vi "basic - Transmit UDP Sampling.vi"() -> ()   [LabVIEW 2020]
uses:
  _controls/comm_computedMAC-IP.ctl
  _controls/comm_udp_tx.ctl
  _controls/comm_config_vl_tx.ctl
  _polimorphicInstances/session/Fdx Create Session (Tx-UDP Port-Oriented).vi
  bsp/AFDX_Transmit/Fdx Create Tx VL.vi
  _polimorphicInstances/udpPort/Fdx Create UDP Port (TX-CommPort).vi
  _polimorphicInstances/control/Fdx Start (Tx).vi
  _polimorphicInstances/control/Fdx Stop (Tx).vi
  _polimorphicInstances/session/Fdx Close Session (Port).vi
  AIM664LV.lvlib
panel:
  out "Duplicated":bool
  in  "VL Config":T1={"VlId"=60, "NumOfSubVl"=2, "rate ms [Bag]"=128, "domainID"=1, "sideID"=1, "locationID"=1, "interfaceID"=1, "NetSelect"=3, "Skew"=0, "MaxFrameLength"=1000, "FrameBufferSize"=0} {"NetSelect" items=["FDX_TX_FRAME_DLY_A"=0, "FDX_TX_FRAME_DLY_B"=1, "FDX_TX_FRAME_BOTH "=3, "FDX_TX_FRAME_ONLY_A"=4, "FDX_TX_FRAME_ONLY_B "=5]; "interfaceID" format="%.0b"}
  in  "CommPort Config":T2[](array[typedef])=[{"PortType"=enum."FDX_UDP_SAMPLING", "partitionID"=1, "SubVlId"=1, "UdpSrcPort"=1, "UdpDstPort"=1, "SampleRateMs"=128.0, "UdpNumBufMessages"=0, "UdpMaxMessageSize"=1000}, {"PortType"=enum."FDX_UDP_SAMPLING", "partitionID"=1, "SubVlId"=2, "UdpSrcPort"=2, "UdpDstPort"=2, "SampleRateMs"=128.0, "UdpNumBufMessages"=0, "UdpMaxMessageSize"=1000}]
  in  "millisecond multiple":u32=128
  in  "PortMap":u32
  out "IndexCycleCount":u32[](array[numeric])
  out "MsgCount":u32[](array[numeric])
  out "CurrentIndex":u32[](array[numeric])
  out "BytesWritten":u32[](array[numeric])
  in  "Port":u32
  in  "Board":u32
  out "current time":timestamp=timestamp(3677762637.591913 s since 1904-01-01)
  out "current irig time":T3={"SignOut"=40, "DayOut"=1, "HourOut"=1, "MinOut"=28, "SecondOut"=39, "MilliSecOut"=539, "MicroSecOut"=300, "NanoSecOut"=0, "InfoOut"=0, "Mode"=3}
  out "CommPort Addresses":T4[](array[typedef]) {"MACsrc" format="%.0x"}
  out "Data to be sent":u8[](array[numeric])=[255, 255, 255, 255, 255, 255, 255, 255, 255, 255, 255, 255, 255, 255, 255, 255, 255, 255, 255, 255, 255, 255, 255, 255, 255, 255, 255, 255, 255, 255, 255, 255, 255, 255, 255, 255, 255, 255, 255, 255, 255, 255, 255, 255, 255, 255, 255, 255, 255, 255, 255, 255, 255, 255, 255, 255, 255, 255, 255, 255, 255, 255, 255, 255, 255, 255, 255, 255, 255, 255, 255, 255, 255, 255, 255, 255, 255, 255, 255, 255, 255, 255, 255, 255, 255, 255, 255, 255, 255, 255, 255, 255, 255, 255, 255, 255, 255, 255, 255, 170] format="%.0x"
  in  "stop":bool
  out "PortInitOut":T5={"PortConfig"=0, "PortUsed"=1, "GlobalMemFree"=0, "SharedMemFree"=0} {"PortConfig" items=["FDX_SINGLE", "FDX_REDUNDANT"]}
  out "error out":errorcluster
  # "ARINC 664 - Transmit UDP - Sampling Port"
  # "Overview: Setup the board to transmit package as UDP using Sampling Port.\n\nRequirement: One AIM ARINC-664 board with installed AIM ARINC 664 BSP.\nRestrictions: None.\nInstruction:\n1. Select the Board ID (0 if you have only one board in your system) and the port number. If you want to validate between two ports in one device, you can use tx board and Rx Board\n2. Run the VI.\n3. See the result in Current IRIG Time"
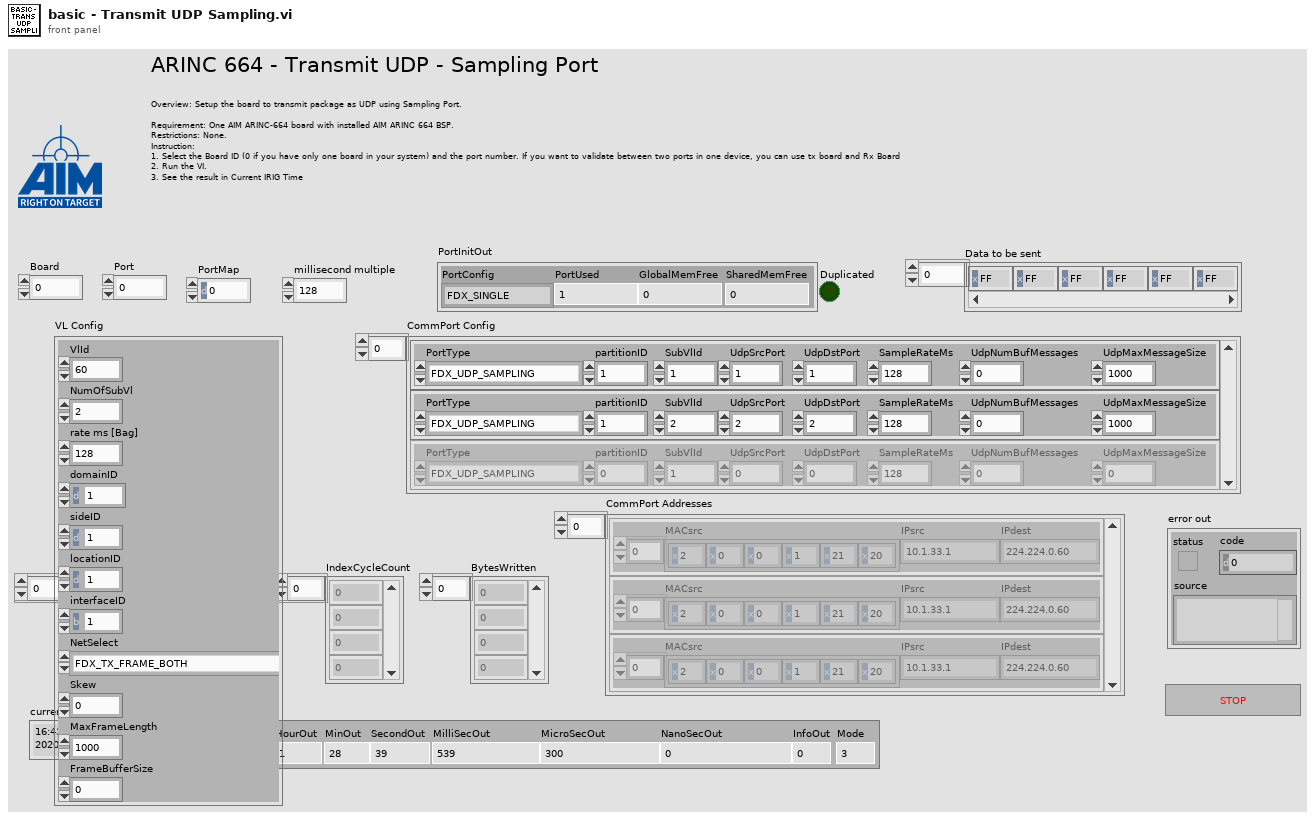
[diagram p1: front panel]
types:
  T1 = typedef "AIM664LV.lvlib/comm_config_vl_tx.ctl" = cluster{"VlId":u16, "NumOfSubVl":u16, "rate ms [Bag]":u32, "domainID":u8, "sideID":u8, "locationID":u8, "interfaceID":u8, "NetSelect":u32, "Skew":u32, "MaxFrameLength":u32, "FrameBufferSize":u32}
  T2 = typedef "AIM664LV.lvlib/comm_udp_tx.ctl" = cluster{"PortType":enum16{"FDX_UDP_SAMPLING", "FDX_UDP_QUEUING"}, "partitionID":u8, "SubVlId":u8, "UdpSrcPort":u16, "UdpDstPort":u16, "SampleRateMs":dbl, "UdpNumBufMessages":u32, "UdpMaxMessageSize":u32}
  T3 = cluster{"SignOut":i32, "DayOut":u32, "HourOut":u32, "MinOut":u32, "SecondOut":u32, "MilliSecOut":u32, "MicroSecOut":u32, "NanoSecOut":u32, "InfoOut":u32, "Mode":u32}
  T4 = typedef "AIM664LV.lvlib/comm_computedMAC-IP.ctl" = cluster{"MACsrc":u8[], "IPsrc":string, "IPdest":string}
  T5 = cluster{"PortConfig":u32, "PortUsed":u32, "GlobalMemFree":u32, "SharedMemFree":u32}
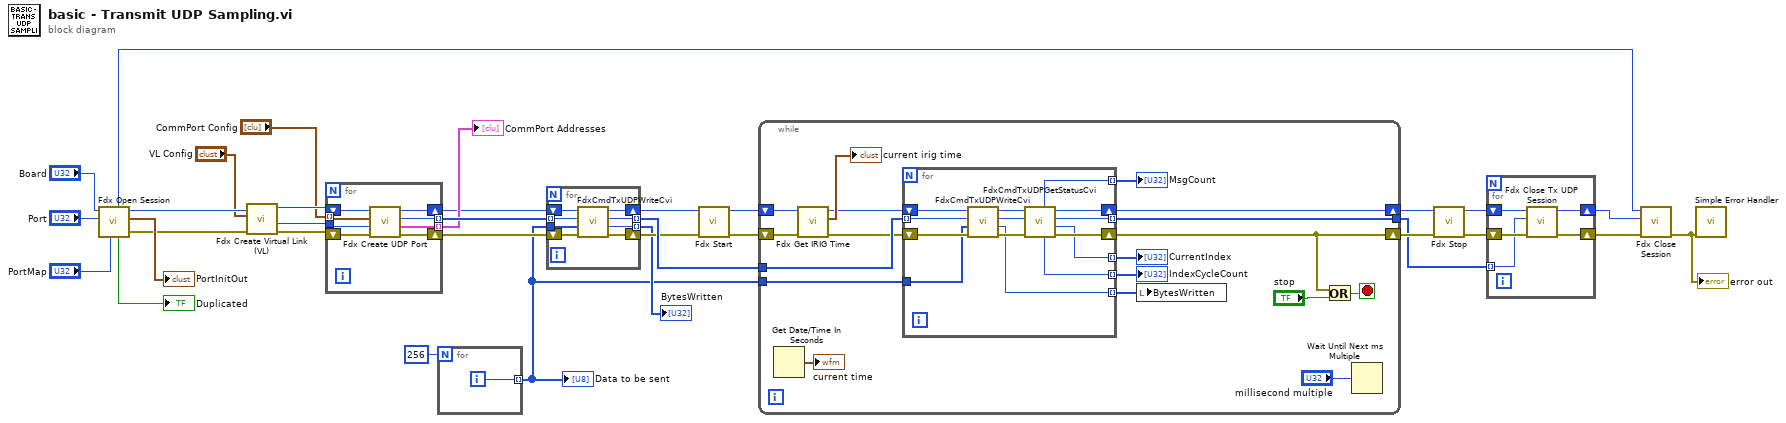
[diagram p0: block diagram]
diagram:
  n1 = call-poly "Fdx Open Session.vi"("PortMap"="PortMap", "port"="Port", "board"="Board") -> ("error out"=w16:errorcluster, "PortInitOut"=→"PortInitOut":T5, "port handle out"=w17:u32, "Duplicated"=→"Duplicated":bool, "InstrumentHandle_board out"=w1:u32)  [unwired: 4 in]
  n2 = call-poly "Fdx Create Virtual Link (VL).vi"("error in (no error)"=w16, "VL Config"="VL Config", "InstrumentHandle in"=w17) -> ("error out"=w14:errorcluster, "VlId"=w13:u16, "InstrumentHandle out"=w15:u32)  [unwired: 6 in]
  n3 = for {
    tunnel: [w40] -> w32 mode=indexing
    tunnel: [w37] -> w29 mode=indexing
    shift-right: [w36] -> w8
    shift-left: w15 -> [w41]
    shift-right: [w39] -> w30
    shift-left: w14 -> [w38]
    tunnel: w13 -> [w35]
    tunnel: "CommPort Config" -> [w34] mode=indexing
    n4 = call-poly "Fdx Create UDP Port.vi"("error in"=w38, "VlId"=w35, "CommPort Config"=w34, "port handle in"=w41) -> ("error out"=w39:errorcluster, "computedAddresses"=w37:T4, "commPort handle out"=w40:u32, "port handle out"=w36:u32)  [unwired: 4 in]
  }
  "CommPort Addresses" <- w29
  n5 = for {
    N: 256 -> [_]
    tunnel: [w42] -> w2 mode=indexing
    i -> [w42]
  }
  "Data to be sent" <- w2
  n6 = for {
    tunnel: w2 -> [w46]
    tunnel: [w48] -> w19 mode=indexing
    shift-right: [w49] -> w27
    shift-left: w30 -> [w50]
    tunnel: w32 -> [w47] mode=indexing
    tunnel: [w43] -> w31 mode=indexing
    shift-right: [w44] -> w7
    shift-left: w8 -> [w45]
    n7 = call "FdxCmdTxUDPWriteCvi.vi"("error in"=w50, "Data"=w46, "UdpHandle"=w47, "InstrumentHandle"=w45) -> ("error out"=w49:errorcluster, "BytesWritten"=w48:u32, "UdpHandleOut"=w43:u32, "InstrumentHandle"=w44:u32)  [unwired: 4 in]
  }
  "BytesWritten" <- w19
  n8 = call-poly "Fdx Start.vi"("error in"=w27, "InstrumentHandle_port in"=w7) -> ("error out"=w26:errorcluster, "InstrumentHandle_port out"=w25:u32)  [unwired: 8 in]
  n9 = while {
    tunnel: w31 -> [w56]
    tunnel: [w61] -> w22
    shift-right: [w52] -> w28
    shift-left: w25 -> [w65]
    tunnel: w2 -> [w51]
    shift-right: [w60] -> w23
    shift-left: w26 -> [w64]
    stop <- w67 stop-if-true
    n10 = Get Date/Time In Seconds() -> (seconds since 1Jan1904=→"current time":timestamp)
    n11 = call "Fdx Get IRIG Time.vi"("error in (no error)"=w64, "InstrumentHandle_board in"=w65) -> ("error out"=w55:errorcluster, "Curent Irig Time"=→"current irig time":T3, "InstrumentHandle_board out"=w53:u32)  [unwired: 7 in]
    n12 = for {
      tunnel: [w69] -> w61 mode=indexing
      tunnel: [w72] -> w59 mode=indexing
      tunnel: [w71] -> w58 mode=indexing
      tunnel: [w73] -> w57 mode=indexing
      tunnel: w56 -> [w81] mode=indexing
      tunnel: [w78] -> w54 mode=indexing
      tunnel: w51 -> [w77]
      shift-right: [w82] -> w60
      shift-left: w55 -> [w80]
      shift-right: [w70] -> w52
      shift-left: w53 -> [w76]
      n13 = call "FdxCmdTxUDPWriteCvi.vi"("error in"=w80, "Data"=w77, "UdpHandle"=w81, "InstrumentHandle"=w76) -> ("error out"=w79:errorcluster, "BytesWritten"=w78:u32, "UdpHandleOut"=w74:u32, "InstrumentHandle"=w75:u32)  [unwired: 4 in]
      n14 = call "FdxCmdTxUDPGetStatusCvi.vi"("error in"=w79, "UdpHandle"=w74, "InstrumentHandle"=w75) -> ("error out"=w82:errorcluster, "CurrentIndex"=w72:u32, "UdpHandleOut"=w69:u32, "InstrumentHandle"=w70:u32, "IndexCycleCount"=w73:u32, "MsgCount"=w71:u32)  [unwired: 3 in]
    }
    "CurrentIndex" <- w59
    "MsgCount" <- w58
    "IndexCycleCount" <- w57
    n15 = local write "BytesWritten"(w54) -> ()
    n16 = Or(x=w60, y="stop") -> (x .or. y?=w67:bool)
    n17 = Wait Until Next ms Multiple(millisecond multiple="millisecond multiple") -> ()  [unwired: 1 out]
  }
  n18 = call-poly "Fdx Stop.vi"("error in"=w23, "InstrumentHandle_port in"=w28) -> ("error out"=w21:errorcluster, "InstrumentHandle_port out"=w6:u32)  [unwired: 8 in]
  n19 = for {
    tunnel: w22 -> [w85] mode=indexing
    shift-right: [w86] -> w20
    shift-left: w21 -> [w87]
    shift-right: [w83] -> w5
    shift-left: w6 -> [w84]
    n20 = call "Fdx Close Tx UDP Session.vi"("error in"=w87, "UdpHandle"=w85, "InstrumentHandle"=w84) -> ("error out"=w86:errorcluster, "InstrumentHandle"=w83:u32)  [unwired: 7 in]
  }
  n21 = call-poly "Fdx Close Session.vi"("error in"=w20, "InstrumentHandle_port in"=w5, "InstrumentHandle_board in"=w1) -> ("error out"=w4:errorcluster)  [unwired: 8 in]
  "error out" <- w4
  n22 = call <vilib>:"Simple Error Handler.vi"("error in (no error)"=w4) -> ()  [unwired: 4 in, 5 out]
